vi "Create_Email_Message.vi"(10 "Responsible Mail":string, 11 "Warning":string) -> ()   [LabVIEW 2016]
panel:
  out "String":string
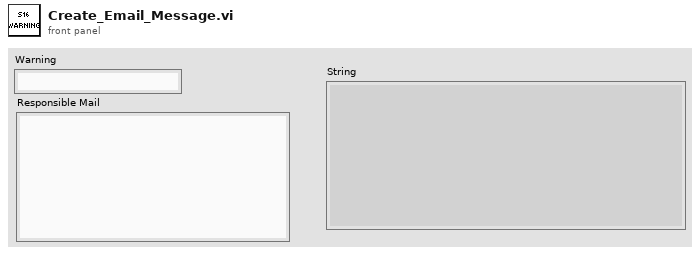
[diagram p1: front panel]
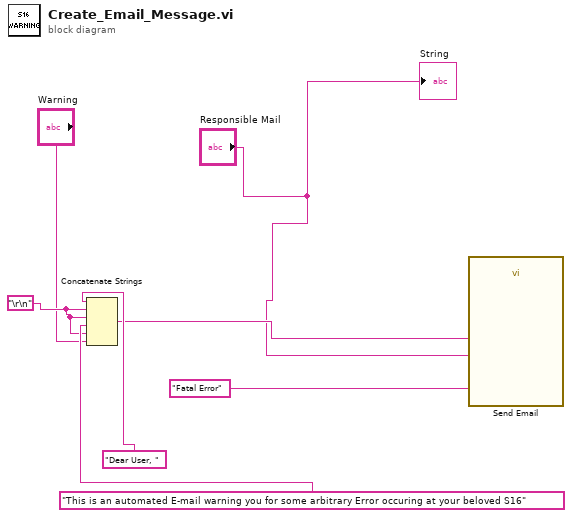
[diagram p0: block diagram]
diagram:
  w3 = "\r\n"
  n1 = Concatenate Strings("Dear User, ", w3, w3, "This is an automated E-mail warning you for some arbitrary Error occuring at your beloved S16", w3, "Warning") -> (w5:string)
  n2 = call "Send Email"("Message"=w5, "Subject"="Fatal Error", "Recipients"="Responsible Mail") -> ()  [unwired: 8 in, 1 out]
  "String" <- "Responsible Mail"
